vi "BuildUpdatePublisherText.vi"(2 "New Publisher":T2, 3 "ROS_Master in":T1) -> (1 "XML":string)   [LabVIEW 2014]
doc: "Builds XML to update publisher"
uses:
  <userlib>/ROS for LabVIEW Software/ROS/Code/ROS_Master/ROS_Topic.ctl
  <userlib>/ROS for LabVIEW Software/ROS/Code/ROS_Master/ROS_Master.ctl
  <userlib>/ROS for LabVIEW Software/ROS/Code/ROS_Master/ROS_Node.ctl
  <userlib>/ROS for LabVIEW Software/ROS/Code/ROS_Master/ROS_Service.ctl
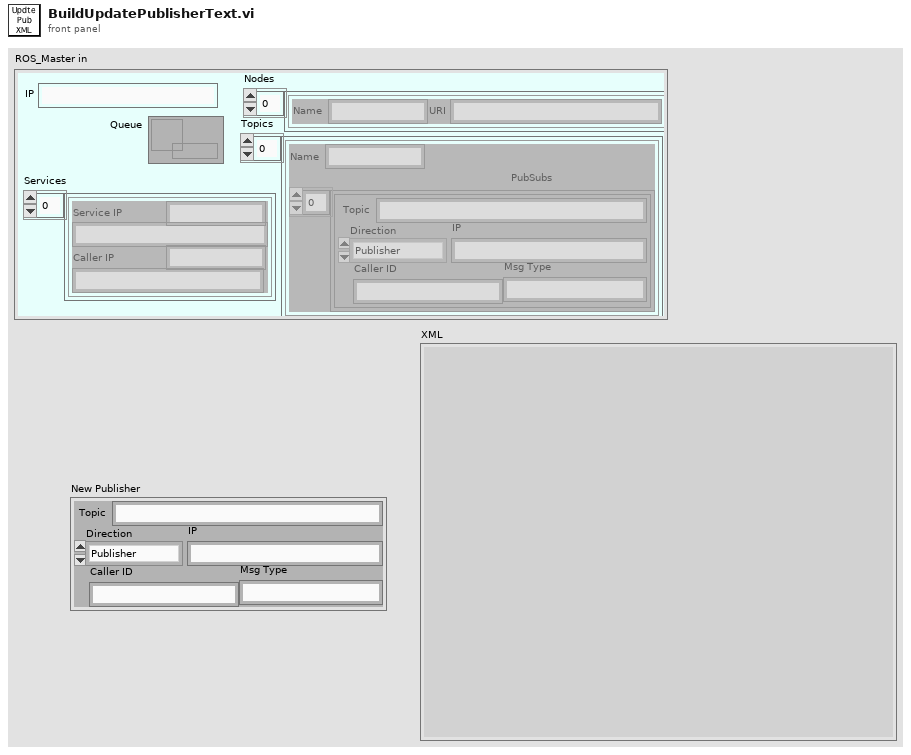
[diagram p1: front panel]
types:
  T1 = typedef "ROS_Master.ctl" = cluster{"IP":string, "Topics":cluster{"Name":string, "PubSubs":T2[]}[], "Nodes":T3[], "Services":T4[], "Queue":refnum<queue>}
  T2 = typedef "ROS_Topic.ctl" = cluster{"Caller ID":string, "IP":string, "Msg Type":string, "Direction":enum16{"Publisher", "Subscriber"}, "Topic":string}
  T3 = typedef "ROS_Node.ctl" = cluster{"Name":string, "URI":string}
  T4 = typedef "ROS_Service.ctl" = cluster{"Service":string, "Service IP":string, "Caller IP":string, "Caller ID":string}
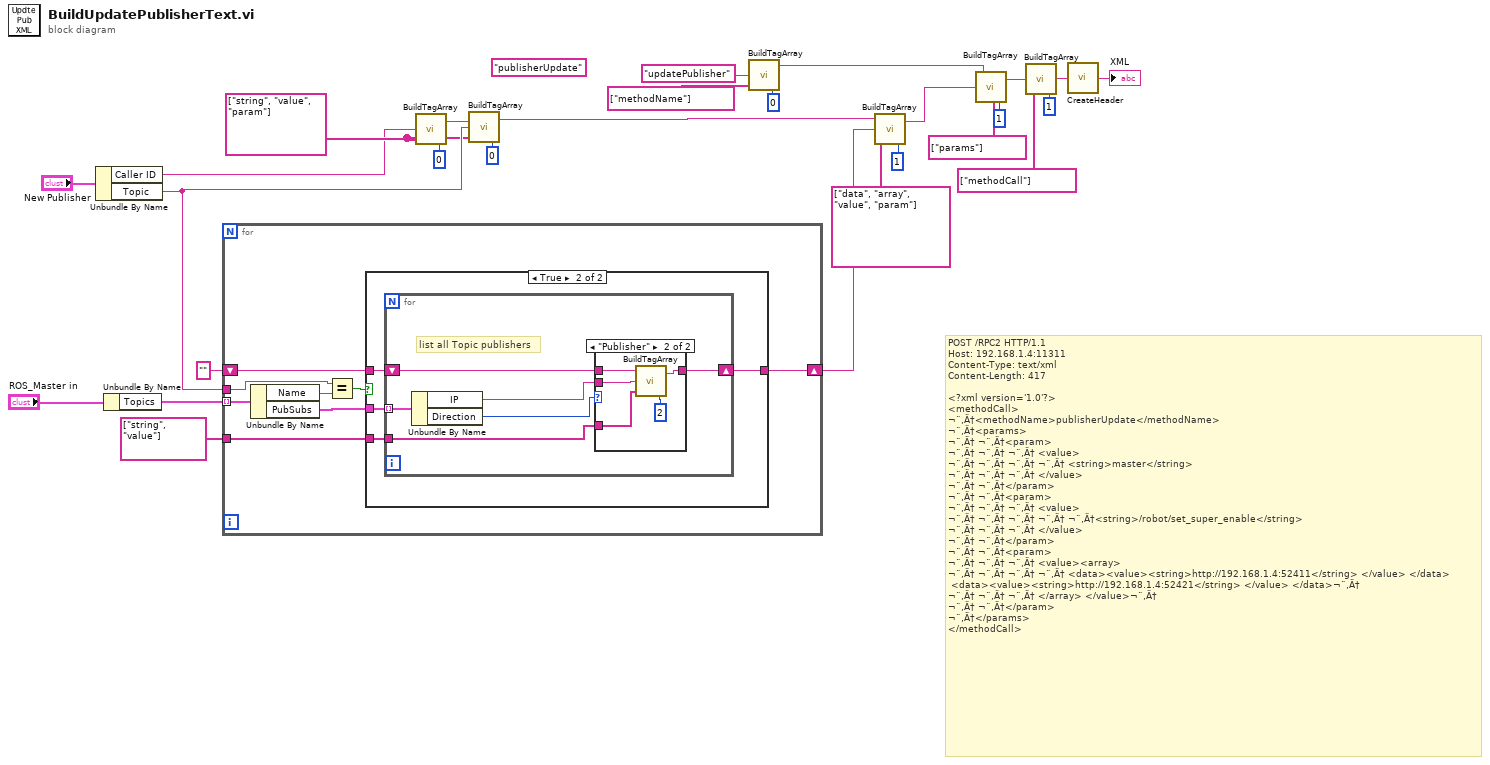
[diagram p0: block diagram]
diagram:
  (unwired) "publisherUpdate" ("value")
  w12 = string[] ["string", "value", "param"] ("tags")
  # "POST /RPC2 HTTP/1.1\nHost: 192.168.1.4:11311\nContent-Type: text/xml\nContent-Length: 417\n\n<?xml version='1.0'?>\n<methodCall>\n¬¨‚Ä†<methodName>publisherUpdate</methodName>\n¬¨‚Ä†<params>\n¬¨‚Ä† ¬¨‚Ä†<param>\n¬¨‚Ä† ¬¨‚Ä† ¬¨‚Ä† <value>\n¬¨‚Ä† ¬¨‚Ä† ¬¨‚Ä† ¬¨‚Ä† <string>master</string>\n¬¨‚Ä† ¬¨‚Ä† ¬¨‚Ä† </value>\n¬¨‚Ä† ¬¨‚Ä†</param>\n¬¨‚Ä† ¬¨‚Ä†<param>\n¬¨‚Ä† ¬¨‚Ä† ¬¨‚Ä† <value>\n¬¨‚Ä† ¬¨‚Ä† ¬¨‚Ä† ¬¨‚Ä† ¬¨‚Ä†<string>/robot/set_super_enable</string>\n¬¨‚Ä† ¬¨‚Ä† ¬¨‚Ä† </value>\n¬¨‚Ä† ¬¨‚Ä†</param>\n¬¨‚Ä† ¬¨‚Ä†<param>\n¬¨‚Ä† ¬¨‚Ä† ¬¨‚Ä† <value><array>\n¬¨‚Ä† ¬¨‚Ä† ¬¨‚Ä† ¬¨‚Ä† <data><value><string>http://192.168.1.4:52411</string> </value> </data>\n\t<data><value><string>http://192.168.1.4:52421</string> </value> </data>¬¨‚Ä†\n¬¨‚Ä† ¬¨‚Ä† ¬¨‚Ä† </array> </value>¬¨‚Ä†\n¬¨‚Ä† ¬¨‚Ä†</param>\n¬¨‚Ä†</params>\n</methodCall>"
  n1 = Unbundle By Name("New Publisher") -> ("Caller ID"=w3:string, "Topic"=w14:string)
  n2 = Unbundle By Name("ROS_Master in") -> ("Topics"=w27:cluster{"Name":string, "PubSubs":T2[]}[])
  n3 = for {
    tunnel: w14 -> [w30]
    tunnel: w27 -> [w35] mode=indexing
    shift-right: [w34] -> w25
    shift-left: "" ("string out") -> [w28]
    tunnel: string[] ["string", "value"] ("tags") -> [w32]
    n4 = Unbundle By Name(w35) -> ("Name"=w29:string, "PubSubs"=w33:T2[])
    n5 = Equal?(x=w30, y=w29) -> (x = y?=w31:bool)
    n6 = case shown="True" w31 {
      tunnel: [w36 w40] -> w34
      tunnel: w33 -> [_ w38]
      tunnel: w32 -> [_ w37]
      tunnel: w28 -> [w36 w39]
      frame False {
      }
      frame True {
        n7 = for {
          shift-right: [w46] -> w40
          shift-left: w39 -> [w43]
          tunnel: w38 -> [w45] mode=indexing
          tunnel: w37 -> [w42]
          # "list all Topic publishers"
          n8 = Unbundle By Name(w45) -> ("IP"=w41:string, "Direction"=w44:enum16{"Publisher", "Subscriber"})
          n9 = case shown="\"Publisher\"" w44 {
            tunnel: [w47 w52] -> w46
            tunnel: w43 -> [w47 w51]
            tunnel: w42 -> [_ w50]
            tunnel: w41 -> [_ w49]
            frame Default {
            }
            frame "Publisher" {
              n10 = call <userlib>:"BuildTagArray.vi"("Indent"=i8 2, "tags"=w50, "value"=w49, "string in"=w51) -> ("string out"=w52:string)
            }
          }
        }
      }
    }
  }
  n11 = call <userlib>:"BuildTagArray.vi"("Indent"=i8 0, "tags"=w12, "value"=w3) -> ("string out"=w4:string)  [unwired: 1 in]
  n12 = call <userlib>:"BuildTagArray.vi"("Indent"=i8 0, "tags"=w12, "value"=w14, "string in"=w4) -> ("string out"=w2:string)
  n13 = call <userlib>:"BuildTagArray.vi"("Indent"=i8 0, "tags"=string[] ["methodName"], "value"="updatePublisher") -> ("string out"=w5:string)  [unwired: 1 in]
  n14 = call <userlib>:"BuildTagArray.vi"("Indent"=i8 1, "tags"=string[] ["data", "array", "value", "param"], "value"=w25, "string in"=w2) -> ("string out"=w1:string)
  n15 = call <userlib>:"BuildTagArray.vi"("Indent"=i8 1, "tags"=string[] ["params"], "value"=w1, "string in"=w5) -> ("string out"=w8:string)
  n16 = call <userlib>:"BuildTagArray.vi"("Indent"=i8 1, "tags"=string[] ["methodCall"], "value"=w8) -> ("string out"=w6:string)  [unwired: 1 in]
  n17 = call <userlib>:"CreateHeader.vi"("Content"=w6) -> ("XML"=→"XML":string)
